vi "Array Element Counter.vi"(10 "Size input":i32[](array[numeric])) -> (2 "Number of Elements":i32)   [LabVIEW 2016]
doc: "This VI takes in an array of sizes (from an greater than 1D array) and counts the number of elements from the multidimensional size."
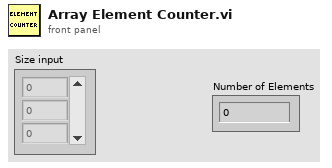
[diagram p1: front panel]
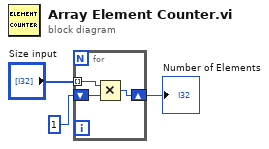
[diagram p0: block diagram]
diagram:
  n1 = for {
    tunnel: "Size input" -> [w6] mode=indexing
    shift-right: [w4] -> w1
    shift-left: 1 -> [w5]
    n2 = Multiply(x=w6, y=w5) -> (x*y=w4:i32)
  }
  "Number of Elements" <- w1
